vi "Run Block Finished.vi"(8 "error in (no error)":errorcluster, 11 "Monkey in":refnum<class "Monkey.lvclass">) -> (0 "error out":errorcluster, 3 "Monkey out":refnum<class "Monkey.lvclass">)   [LabVIEW 2020, in "CIRCUS_uServices.lvlib" / "Monkey.lvlib" / "Monkey.lvclass"]
doc: "Indicate that the Run Block has finished (set the Running flag to False)"
uses:
  Monkey.lvclass
  Monkey.lvclass/Monkey.ctl
  Run Utilities/Run Block/Run Block.lvclass
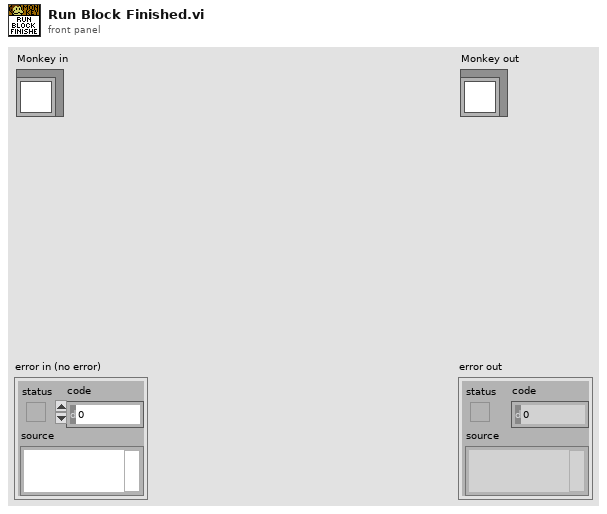
[diagram p1: front panel]
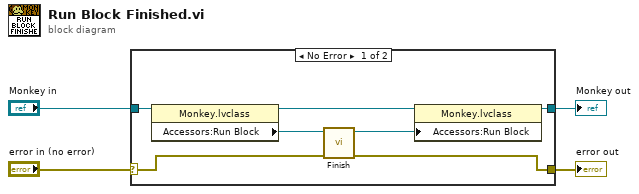
[diagram p0: block diagram]
diagram:
  n1 = case shown="No Error" "error in (no error)" {
    selector: "error in (no error)" -> [w6 w13]
    tunnel: [w5 w13] -> w3
    tunnel: [w9 w12] -> w1
    tunnel: "Monkey in" -> [w11 w12]
    frame No Error {
      n2 = property class="Monkey.lvclass"(reference=w11) -> (reference out=w10:refnum<class "Monkey.lvclass">, "Accessors:Run Block"=w8:refnum<class "Run Block.lvclass">)  [unwired: 1 in, 1 out]
      n3 = call-dynamic "Finish.vi"("error in (no error)"=w6, "Run Block in"=w8) -> ("error out"=w5:errorcluster, "Run Block out"=w7:refnum<class "Run Block.lvclass">)  [unwired: 8 in]
      n4 = property class="Monkey.lvclass"(reference=w10, "Accessors:Run Block"=w7) -> (reference out=w9:refnum<class "Monkey.lvclass">)  [unwired: 1 in, 1 out]
    }
    frame Error {
    }
  }
  "error out" <- w3
  "Monkey out" <- w1
